vi "PrefDialog.vi"(8 "error in (no error)":errorcluster, 11 "MyPluginsBase in":refnum<class "Simulation.lvclass">) -> (0 "error out":errorcluster, 3 "MyPluginsBase out":refnum<class "Simulation.lvclass">)   [LabVIEW 2018, in "DigitizerPlugins.lvlib" / "Simulation.lvclass"]
uses:
  Simulation.lvclass
  F:/Projects/ICDAS/NistPluggableModules/Digitizer/DigitizerPlugins/DigitizerBaseClass/DigitizerBase.lvclass
  F:/Program Files (x86)/National Instruments/LabVIEW 2018/user.lib/NIST/BaseClasses/BasePlugin_class/BasePlugin.lvclass
  DigitizerBaseClass/Typedefs/Acquisition.ctl
  DigitizerBaseClass/Typedefs/Channel.ctl
  DigitizerBaseClass/Typedefs/Trigger.ctl
  DigitizerBaseClass/Typedefs/TrigSource.ctl
  DigitizerBaseClass/DigitizerBase.lvclass/DigitizerBase.ctl
  <userlib>/NIST/BaseClasses/BasePlugin_class/BasePlugin.lvclass/BasePlugin.ctl
  Simulation.lvclass/Simulation.ctl
  DigitizerBaseClass/Accessors/Write Acquisition.vi
  DigitizerBaseClass/Accessors/Write Trigger.vi
  DigitizerBaseClass/Accessors/Write Channels.vi
  <userlib>/NIST/BaseClasses/BasePlugin_class/Accessors/Read PluginIniFilePath.vi
  Accessors/Read Function.vi
  Accessors/Write Function.vi
  DigitizerBaseClass/Accessors/Read Acquisition.vi
  DigitizerBaseClass/Accessors/Read Channels.vi
  DigitizerBaseClass/Accessors/Read Trigger.vi
  FGen/MemberClasses/FunctionBaseClass/FunctionBase.lvclass
  <vilib>/Utility/config.llb/NI_LVConfig.lvlib
  <userlib>/NIST/NISTErrorLib/NISTErrorLib.lvlib
  DigitizerBaseClass/DigitizerBase.lvclass
panel:
  in  "btnFuncConfig":bool
  in  "btnCancel":bool
  in  "btnDone":bool
  in  "Trigger":T1
  in  "Channels":T3[](array[typedef])
  in  "Acquisition":T4 {"SampleMode" items=["Real Time", "Equivalent Time"]}
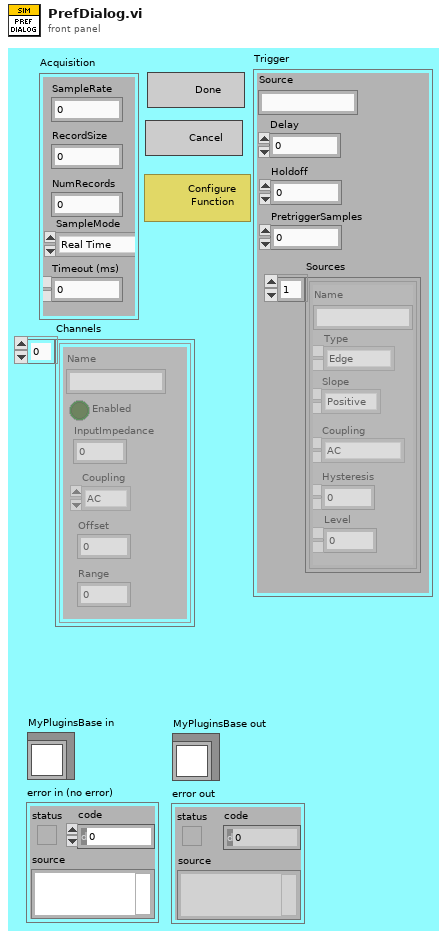
[diagram p1: front panel]
types:
  T1 = typedef "DigitizerPlugins.lvlib/DigitizerBase.lvclass/Trigger.ctl" = cluster{"Source":string, "Delay":dbl, "Holdoff":dbl, "PretriggerSamples":i32, "Sources":T2[]}
  T2 = typedef "DigitizerPlugins.lvlib/DigitizerBase.lvclass/TrigSource.ctl" = cluster{"Name":string, "Coupling":enum16{"AC", "DC", "HF Reject", "LF Reject", "Noise Reject"}, "Hysteresis":dbl, "Level":dbl, "Slope":enum16{"Positive", "Negative"}, "Type":enum16{"Edge", "Width", "Runt", "Glitch", "TV", "Window"}}
  T3 = typedef "DigitizerPlugins.lvlib/DigitizerBase.lvclass/Channel.ctl" = cluster{"Name":string, "Enabled":bool, "InputImpedance":dbl, "Coupling":enum16{"AC", "DC", "Gnd"}, "Offset":dbl, "Range":dbl}
  T4 = typedef "DigitizerPlugins.lvlib/DigitizerBase.lvclass/Acquisition.ctl" = cluster{"SampleRate":dbl, "RecordSize":i32, "NumRecords":i32, "SampleMode":i32, "Timeout (ms)":i32}
  T5 = enum32{"Invalid", "Default", "Floating", "Floating/Auto-Hide", "Modal"}
  T6 = typedef "NI_LVConfig.lvlib/Config Data RefNum.ctl" = refnum<k1>
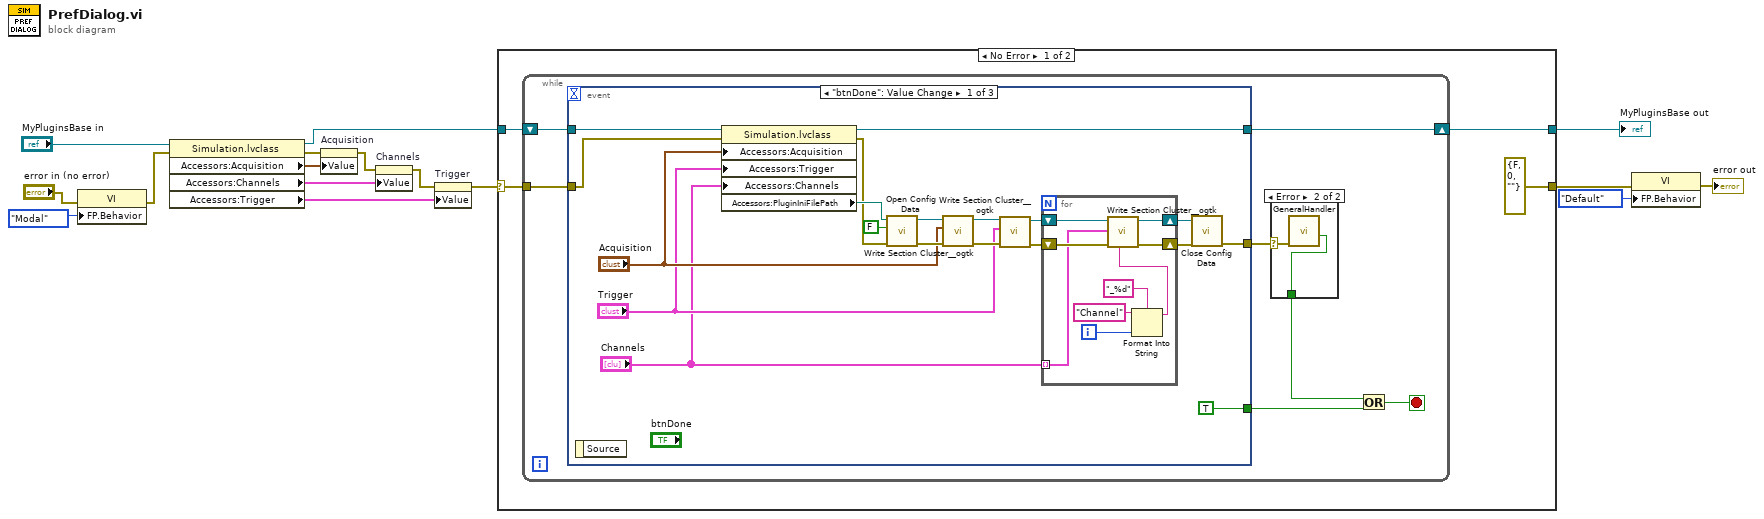
[diagram p0: block diagram]
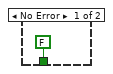
[diagram p2: hidden frame]
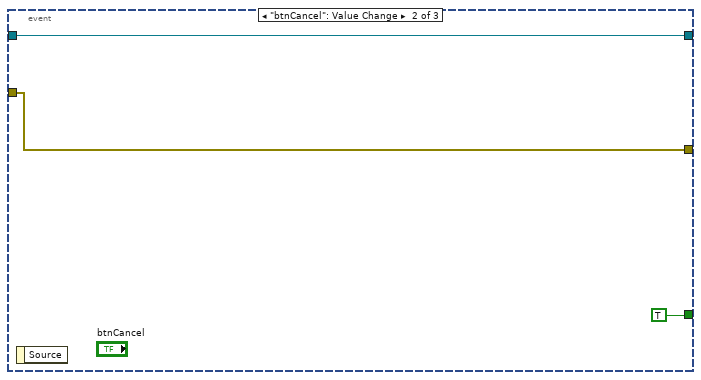
[diagram p3: hidden frame]
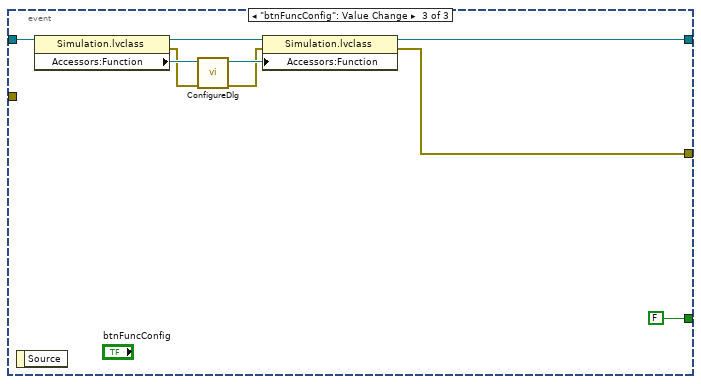
[diagram p4: hidden frame]
diagram:
  n1 = property class="VI"(error in="error in (no error)", "FP.Behavior"=T5."Modal" ("Front Panel Window:Behavior")) -> (error out=w14:errorcluster)  [unwired: 1 in, 1 out]
  n2 = property class="Simulation.lvclass"(reference="MyPluginsBase in", error in=w14) -> (reference out=w5:refnum<class "Simulation.lvclass">, error out=w11:errorcluster, "Accessors:Acquisition"=w12:T4, "Accessors:Channels"=w10:T3[], "Accessors:Trigger"=w8:T1)
  n3 = property on="Acquisition" class="Clust (strict)"(error in=w11, "Value"=w12) -> (error out=w9:errorcluster)  [unwired: 1 in, 1 out]
  n4 = property on="Channels" class="Arr (strict)"(error in=w9, "Value"=w10) -> (error out=w7:errorcluster)  [unwired: 1 in, 1 out]
  n5 = property on="Trigger" class="Clust (strict)"(error in=w7, "Value"=w8) -> (error out=w6:errorcluster)  [unwired: 1 in, 1 out]
  n6 = case shown="No Error" w6 {
    selector: w6 -> [w19 w72]
    tunnel: w5 -> [w20 w71]
    tunnel: [w18 w71] -> w4
    tunnel: [errorcluster {"status"=FALSE, "code"=0, "source"=""} ("error IO") w72] -> w3
    frame No Error {
      n7 = while {
        shift-right: [w21] -> w18
        shift-left: w20 -> [w27]
        tunnel: w19 -> [w26]
        stop <- w22 stop-if-true
        n8 = event shown="[0] \"btnDone\": Value Change" {
          selector: _ -> [_ _ _]
          dyn-events: _ -> [_ _ _]
          timeout: _ -> [_ _ _]
          tunnel: w27 -> [w49 w61 w70]
          tunnel: w26 -> [w48 w60 _]
          tunnel: [w35 w60 w63] -> w25
          tunnel: [TRUE TRUE FALSE] -> w24
          tunnel: [w33 w61 w64] -> w21
          event "btnDone": Value Change {
            n9 = event-data() -> ()  [unwired: 1 in, 1 out]
            n10 = property class="Simulation.lvclass"(reference=w49, error in=w48, "Accessors:Acquisition"="Acquisition", "Accessors:Trigger"="Trigger", "Accessors:Channels"="Channels") -> (reference out=w33:refnum<class "Simulation.lvclass">, error out=w46:errorcluster, "Accessors:PluginIniFilePath"=w47:path)
            n11 = call <vilib>:"Open Config Data.vi"("error in (no error)"=w46, "create file if necessary (T)"=FALSE, "configuration file path"=w47) -> ("error out"=w43:errorcluster, "refnum"=w44:T6)  [unwired: 6 in, 1 out]
            n12 = call <userlib>:"Write Section Cluster__ogtk.vi"("error in (no error)"=w43, "Section Formatted Cluster"="Acquisition", "refnum"=w44) -> ("error out"=w40:errorcluster, "dup refnum"=w41:T6)  [unwired: 7 in]
            n13 = call <userlib>:"Write Section Cluster__ogtk.vi"("error in (no error)"=w40, "Section Formatted Cluster"="Trigger", "refnum"=w41) -> ("error out"=w32:errorcluster, "dup refnum"=w31:T6)  [unwired: 7 in]
            n14 = for {
              shift-right: [w56] -> w36
              shift-left: w32 -> [w58]
              shift-right: [w55] -> w37
              shift-left: w31 -> [w57]
              tunnel: "Channels" -> [w51] mode=indexing
              i -> [w52]
              n15 = Format Into String(format string="_%d", initial string="Channel", w52) -> (resulting string=w50:string)  [unwired: 1 in, 1 out]
              n16 = call <userlib>:"Write Section Cluster__ogtk.vi"("section (optional)"=w50, "error in (no error)"=w58, "Section Formatted Cluster"=w51, "refnum"=w57) -> ("error out"=w56:errorcluster, "dup refnum"=w55:T6)  [unwired: 6 in]
            }
            n17 = call <vilib>:"Close Config Data.vi"("error in (no error)"=w36, "refnum"=w37) -> ("error out"=w35:errorcluster)  [unwired: 8 in, 1 out]
          }
          event "btnCancel": Value Change {
            n18 = event-data() -> ()  [unwired: 1 in, 1 out]
          }
          event "btnFuncConfig": Value Change {
            n19 = event-data() -> ()  [unwired: 1 in, 1 out]
            n20 = property class="Simulation.lvclass"(reference=w70) -> (reference out=w67:refnum<class "Simulation.lvclass">, error out=w68:errorcluster, "Accessors:Function"=w69:refnum<class "FunctionBase.lvclass">)  [unwired: 1 in]
            n21 = call-dynamic "ConfigureDlg.vi"("error in (no error)"=w68, "FunctionBase in"=w69) -> ("error out"=w65:errorcluster, "FunctionBase out"=w66:refnum<class "FunctionBase.lvclass">)  [unwired: 7 in, 1 out]
            n22 = property class="Simulation.lvclass"(reference=w67, error in=w65, "Accessors:Function"=w66) -> (reference out=w64:refnum<class "Simulation.lvclass">, error out=w63:errorcluster)
          }
        }
        n23 = case shown="Error" w25 {
          selector: w25 -> [_ w29]
          tunnel: [FALSE ("Stop") w30] -> w23
          frame No Error {
          }
          frame Error {
            n24 = call <userlib>:"GeneralHandler.vi"("error in (no error)"=w29) -> ("Stop"=w30:bool)  [unwired: 6 in, 4 out]
          }
        }
        n25 = Or(x=w23, y=w24) -> (x .or. y?=w22:bool)
      }
    }
    frame Error {
    }
  }
  "MyPluginsBase out" <- w4
  n26 = property class="VI"(error in=w3, "FP.Behavior"=T5."Default" ("Front Panel Window:Behavior")) -> (error out=→"error out":errorcluster)  [unwired: 1 in, 1 out]
